vi "Test SG02P2 und G05P1.vi"() -> ()   [LabVIEW 2009]
uses:
  LV-BME Interface/ChnlSettings.ctl
  LV-BME Interface/BME_DG_TriggerSettings.ctl
  DG Classes/BME_DG_System/UpdateChnlTask.ctl
  DG Classes/BME_DG_G05P2/SG05P2 Clock and Trigger Settings.ctl
  LV-BME Interface/ClockSource.ctl
  DG Classes/BME_DG_System/BME_DG_System.lvclass
  ChnlParam.ctl
  DG Classes/BME_DG_Base/BME_DG_Base.lvclass
  DG Classes/BME_DG_Chnl/BME_DG_Chnl.lvclass
  POLARIS BME DG.lvlib
panel:
  in  "Karten Parameter":T1[](array[typedef])=[{"Trigger"={"InputTerminated?"=FALSE, "InternalClockPeriode(µs)"=1000000.0, "TriggerLevel"=1.25, "PresetValue"=0, "DivideBy"=1, "Clock Source"=1, "Gate Divider"=1, "PositiveGate?"=TRUE, "InternalTrigger?"=TRUE, "InternalArm?"=FALSE, "SWTrigger?"=FALSE, "RisingEdge?"=FALSE, "StopOnPreset?"=FALSE, "ResetWhenDone?"=TRUE, "TriggerEnabled?"=TRUE}, "ClockSource "=1, "V2 Trigger"={"Gate Type"=TRUE, "Synchronize Gate"=FALSE, "Force Trigger (µs)"=0.0, "MS Bus"=16}, " prescaller crst oscill."=8, "CardName"="Master"}, {"Trigger"={"InputTerminated?"=TRUE, "InternalClockPeriode(µs)"=0.0, "TriggerLevel"=1.25, "PresetValue"=0, "DivideBy"=1, "Clock Source"=3, "Gate Divider"=1, "PositiveGate?"=TRUE, "InternalTrigger?"=FALSE, "InternalArm?"=FALSE, "SWTrigger?"=FALSE, "RisingEdge?"=FALSE, "StopOnPreset?"=FALSE, "ResetWhenDone?"=FALSE, "TriggerEnabled?"=FALSE}, "ClockSource "=4, "V2 Trigger"={"Gate Type"=TRUE, "Synchronize Gate"=FALSE, "Force Trigger (µs)"=0.0, "MS Bus"=16}, " prescaller crst oscill."=1, "CardName"="S1"}, {"Trigger"={"InputTerminated?"=TRUE, "InternalClockPeriode(µs)"=0.0, "TriggerLevel"=1.25, "PresetValue"=0, "DivideBy"=1, "Clock Source"=3, "Gate Divider"=1, "PositiveGate?"=TRUE, "InternalTrigger?"=FALSE, "InternalArm?"=FALSE, "SWTrigger?"=FALSE, "RisingEdge?"=FALSE, "StopOnPreset?"=FALSE, "ResetWhenDone?"=FALSE, "TriggerEnabled?"=TRUE}, "ClockSource "=1, "V2 Trigger"={"Gate Type"=TRUE, "Synchronize Gate"=FALSE, "Force Trigger (µs)"=0.0, "MS Bus"=16}, " prescaller crst oscill."=1, "CardName"="S2"}] {"V2 Trigger"."MS Bus" format="%04x" items=["Local Primary"=1, "Local Secondary"=2, "Local Force"=4, "Resynchronize"=8, "Master Primary"=16, "Master Secondary"=32, "Master Force"=64, "System Clock"=128, "Delay Clock"=256, "Inhibit Local"=512, "Start Local"=1024, "Start Bus"=2048, "Step Back Local"=4096, "Step Back Bus"=8192, "Enable From E"=65536, "Enable From F"=131072, "Enable From Bus"=262144]; "V2 Trigger"."Force Trigger (µs)" min=0.0 format="%.6f"; "ClockSource" items=["Internal Oscillator"=1, "External Trigger"=2, "Trigger & Oscillator"=3, "MasterSlave Bus"=4]; "Trigger"."Gate Divider" min=1 max=1000000; "Trigger"."Clock Source" items=["Internal Oscillator"=1, "External Trigger"=2, "Trigger & Oscillator"=3]; "Trigger"."InternalClockPeriode(µs)" format="%#_11g"}
  out "Problem Chnls out":string[](array[string])
  out "DelayFormulas":string[](array[string])
  in  "Reset Error":bool
  out "error out":errorcluster
  in  "Update Delay formula":bool=TRUE
  in  "DelayFormula":string="MasterSG02P2_ChnlT0 + 100"
  in  "Aknowledge interrupts":bool
  in  "stop 3":bool=TRUE
  in  "SetDelay":bool=TRUE
  in  "UpdateChnl":bool=TRUE
  in  "ChnlParameter":T4 {"ChnParam2write"."Delay (µs)" min=0.0 max=100000000.0 format="%.5f"}
  out "CountsRemains":i32
  out "TriggerCounters":i32[](array[numeric])
  out "Interrupts":u32[](array[numeric]) format="%b"
  out "RemainingTriggers":T6(array[cluster])=[[{"Time Stamp"=timestamp(3416308194.6875 s since 1904-01-01), "Numeric"=-64}, {"Time Stamp"=timestamp(3416308194.6875 s since 1904-01-01), "Numeric"=4}, {"Time Stamp"=timestamp(3416308194.6875 s since 1904-01-01), "Numeric"=-64}, {"Time Stamp"=timestamp(3416308194.6875 s since 1904-01-01), "Numeric"=-64}], [{"Time Stamp"=timestamp(3416308194.6875 s since 1904-01-01), "Numeric"=-64}, {"Time Stamp"=timestamp(3416308194.6875 s since 1904-01-01), "Numeric"=-64}, {"Time Stamp"=timestamp(3416308194.6875 s since 1904-01-01), "Numeric"=-64}, {"Time Stamp"=timestamp(3416308194.6875 s since 1904-01-01), "Numeric"=-64}], [{"Time Stamp"=timestamp(3416308194.6875 s since 1904-01-01), "Numeric"=-64}, {"Time Stamp"=timestamp(3416308194.6875 s since 1904-01-01), "Numeric"=-64}, {"Time Stamp"=timestamp(3416308194.6875 s since 1904-01-01), "Numeric"=-64}, {"Time Stamp"=timestamp(3416308194.6875 s since 1904-01-01), "Numeric"=-64}]] {"Time Stamp" format="%<%I:%M:%S%3u %p>T"}
  in  "stop 2":bool=TRUE
  in  "ReadStatus":bool=TRUE
  in  "Activate":bool
  in  "ResetModuloCounters":bool=TRUE
  in  "TriggerModulo":u32=4
  out "Modulo Settings":u32[](array[numeric])
  out "Chnls":T5[](array[typedef])=[{" Delay (µs)"=0.0, "On? (false)"=TRUE, "PositiveVoltage?"=TRUE, "50OhmTerminated? "=TRUE, "25OhmOutput?"=FALSE}, {" Delay (µs)"=0.0, "On? (false)"=TRUE, "PositiveVoltage?"=TRUE, "50OhmTerminated? "=TRUE, "25OhmOutput?"=FALSE}, {" Delay (µs)"=0.0, "On? (false)"=TRUE, "PositiveVoltage?"=TRUE, "50OhmTerminated? "=TRUE, "25OhmOutput?"=FALSE}] {"Delay (µs)" min=0.0 max=100000000.0 format="%.5f"}
  in  "Trigger Base":T2={"InputTerminated?"=FALSE, "InternalClockPeriode(µs)"=1000000.0, "TriggerLevel"=1.25, "PresetValue"=0, "DivideBy"=1, "Clock Source"=1, "Gate Divider"=1, "PositiveGate?"=TRUE, "InternalTrigger?"=FALSE, "InternalArm?"=FALSE, "SWTrigger?"=FALSE, "RisingEdge?"=FALSE, "StopOnPreset?"=FALSE, "ResetWhenDone?"=TRUE, "TriggerEnabled?"=TRUE} {"Gate Divider" min=1 max=1000000; "Clock Source" items=["Internal Oscillator"=1, "External Trigger"=2, "Trigger & Oscillator"=3]; "InternalClockPeriode(µs)" format="%#_11g"}
  in  "Selected Chnl":u16(ring) items=["T2", "A2", "B2"]
  in  "Selected Card":u16(ring)=1 items=["Master", "S1", "S2"]
  in  "STOP":bool=TRUE
  in  "ChnParam2write":T5={" Delay (µs)"=0.0, "On? (false)"=TRUE, "PositiveVoltage?"=TRUE, "50OhmTerminated? "=TRUE, "25OhmOutput?"=FALSE} {"Delay (µs)" min=0.0 max=100000000.0 format="%.5f"}
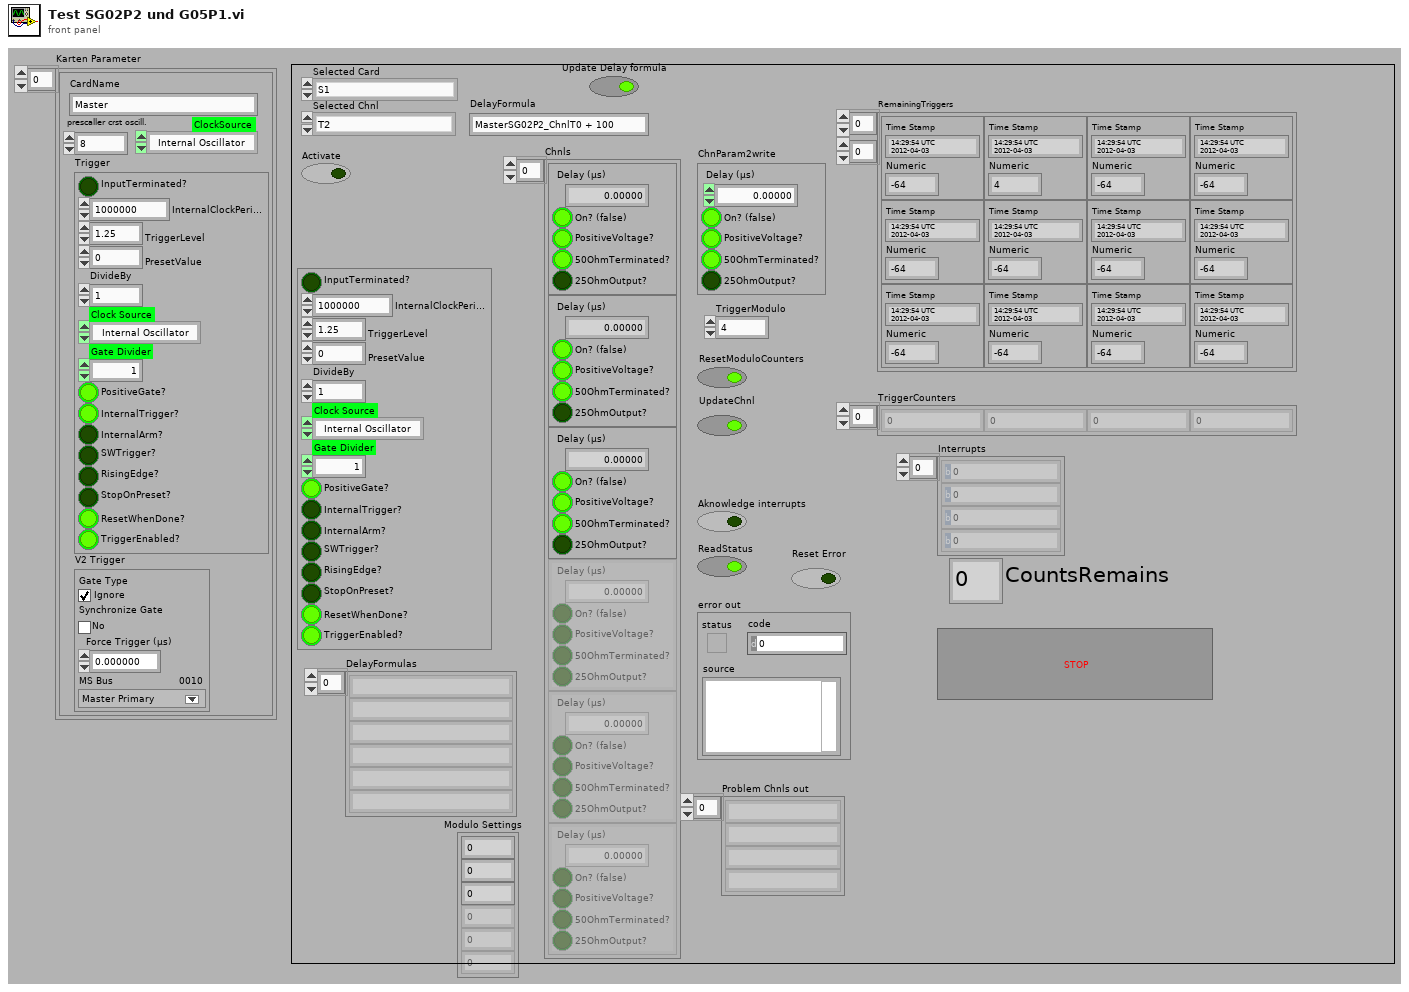
[diagram p1: front panel]
types:
  T1 = typedef "SG05P2 Clock and Trigger Settings.ctl" = cluster{"Trigger":T2, "ClockSource ":T3, "V2 Trigger":cluster{"Gate Type":bool, "Synchronize Gate":bool, "Force Trigger (µs)":dbl, "MS Bus":u32}, " prescaller crst oscill.":u32, "CardName":string}
  T2 = typedef "POLARIS BME DG.lvlib/BME_DG_TriggerSettings.ctl" = cluster{"InputTerminated?":bool, "InternalClockPeriode(µs)":dbl, "TriggerLevel":dbl, "PresetValue":i32, "DivideBy":i32, "Clock Source":u32, "Gate Divider":i32, "PositiveGate?":bool, "InternalTrigger?":bool, "InternalArm?":bool, "SWTrigger?":bool, "RisingEdge?":bool, "StopOnPreset?":bool, "ResetWhenDone?":bool, "TriggerEnabled?":bool}
  T3 = typedef "POLARIS BME DG.lvlib/ClockSource.ctl" = i32
  T4 = typedef "POLARIS BME DG.lvlib/UpdateChnlTask.ctl" = cluster{"ChnlName":string, "ChnParam2write":T5, "TriggerModulo":u32}
  T5 = typedef "POLARIS BME DG.lvlib/ChnlSettings.ctl" = cluster{" Delay (µs)":dbl, "On? (false)":bool, "PositiveVoltage?":bool, "50OhmTerminated? ":bool, "25OhmOutput?":bool}
  T6 = cluster{"Time Stamp":timestamp, "Numeric":i32}[][]
  T7 = typedef "ChnlParam.ctl" = cluster{"ChnlName":string, "DelayFormula":string, "OutputModulo":i32}
  T8 = enum8{"Enabled", "Disabled", "Disabled and Grayed Out"}
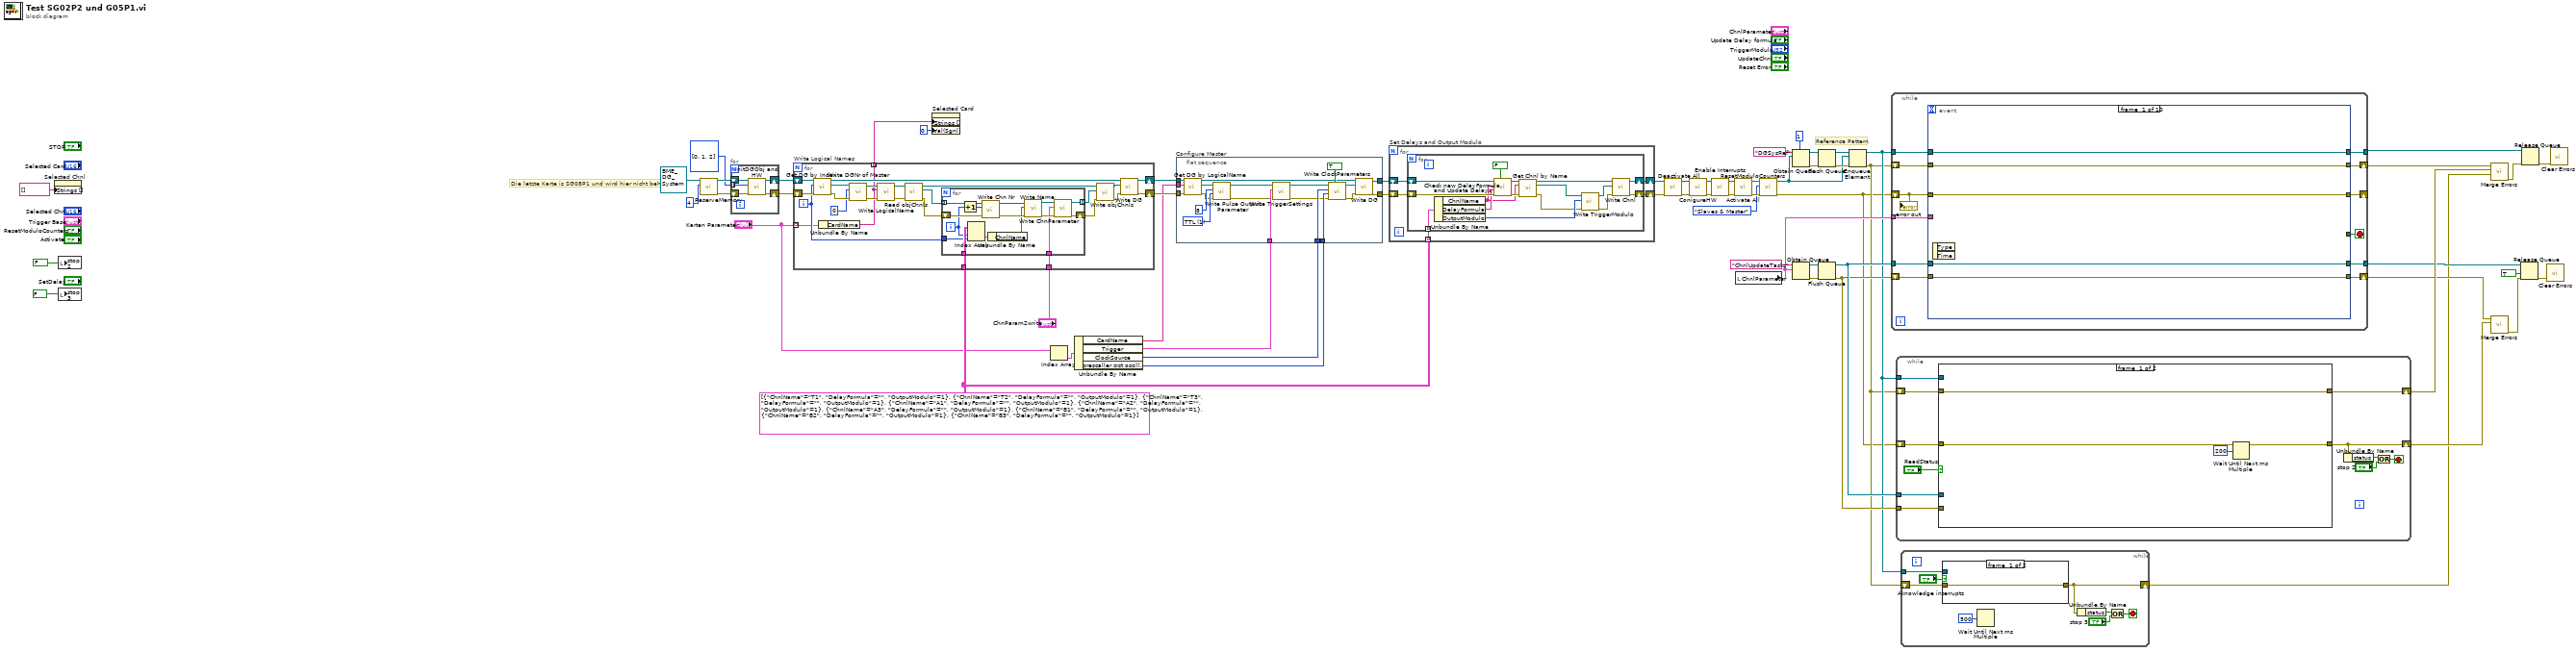
[diagram p0: block diagram]
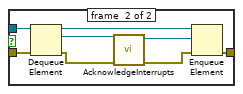
[diagram p2: hidden frame]
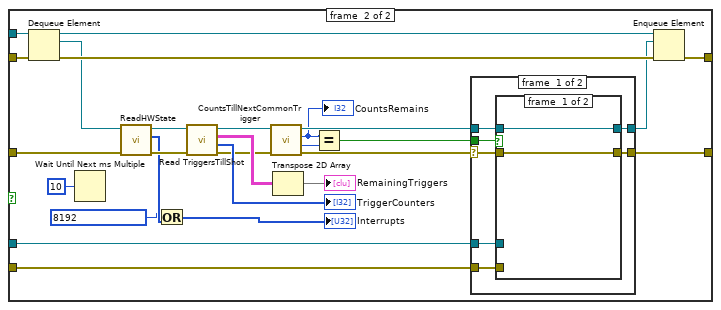
[diagram p3: hidden frame]
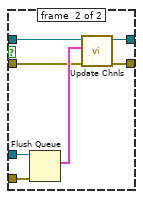
[diagram p4: hidden frame]
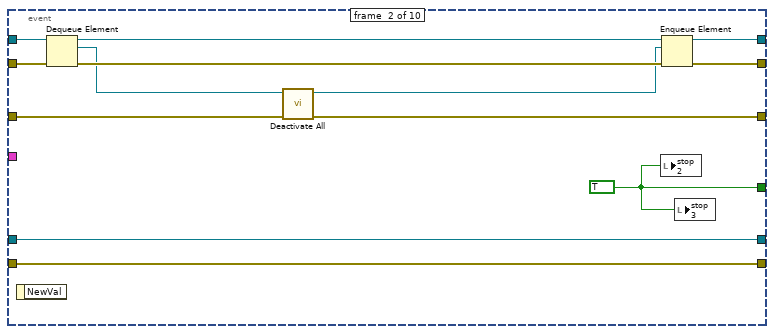
[diagram p6: hidden frame]
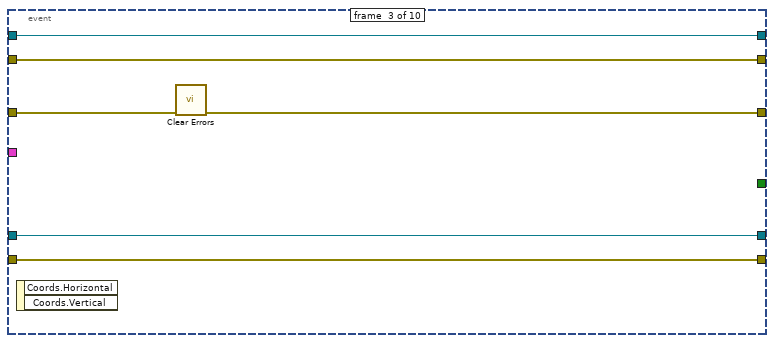
[diagram p7: hidden frame]
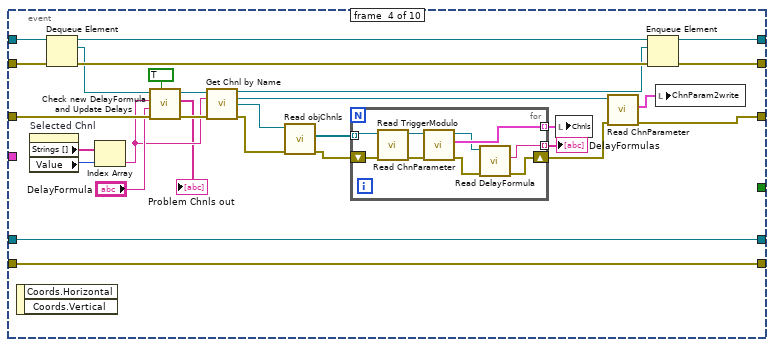
[diagram p8: hidden frame]
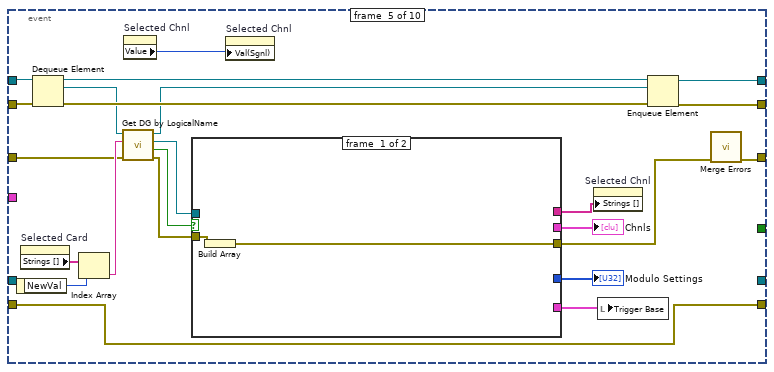
[diagram p9: hidden frame]
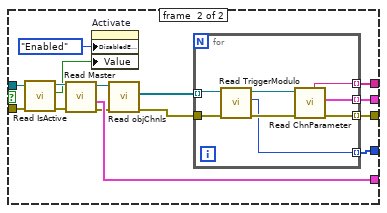
[diagram p10: hidden frame]
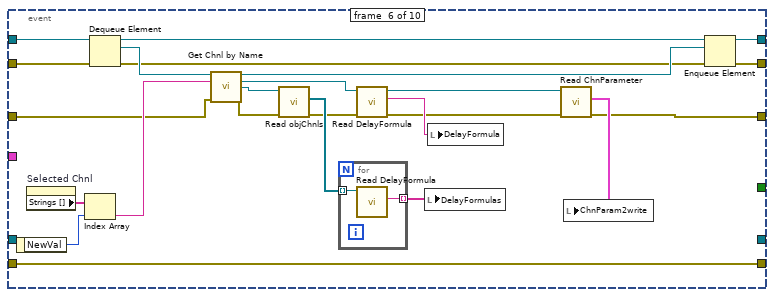
[diagram p11: hidden frame]
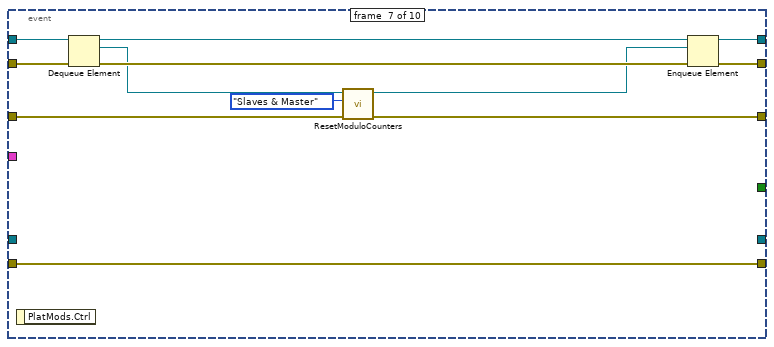
[diagram p12: hidden frame]
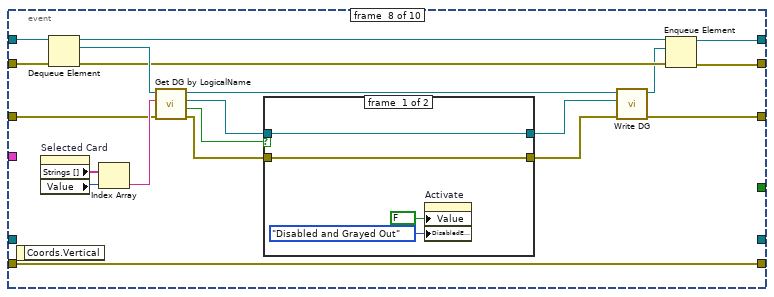
[diagram p13: hidden frame]
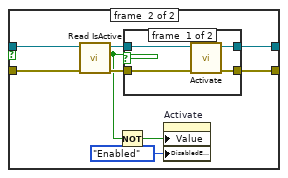
[diagram p14: hidden frame]
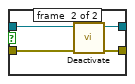
[diagram p15: hidden frame]
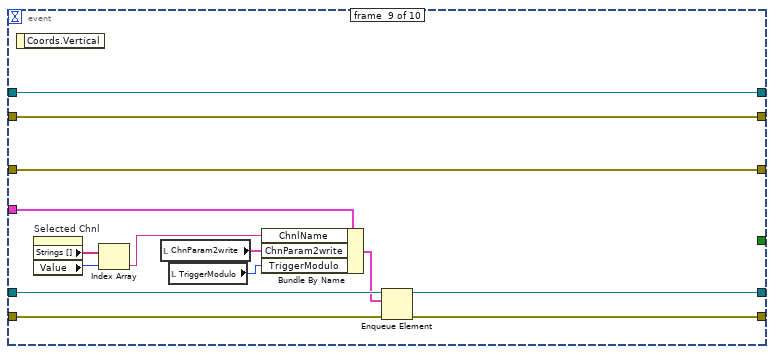
[diagram p16: hidden frame]
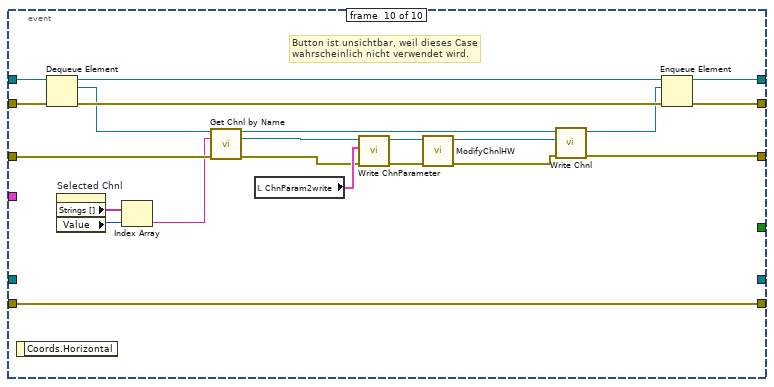
[diagram p17: hidden frame]
diagram:
  w20 = T7[][] [[{"ChnlName"="T1", "DelayFormula"="", "OutputModulo"=1}, {"ChnlName"="T2", "DelayFormula"="", "OutputModulo"=1}, {"ChnlName"="T3", "DelayFormula"="", "OutputModulo"=1}], [{"ChnlName"="A1", "DelayFormula"="", "OutputModulo"=1}, {"ChnlName"="A2", "DelayFormula"="", "OutputModulo"=1}, {"ChnlName"="A3", "DelayFormula"="", "OutputModulo"=1}], [{"ChnlName"="B1", "DelayFormula"="", "OutputModulo"=1}, {"ChnlName"="B2", "DelayFormula"="", "OutputModulo"=1}, {"ChnlName"="B3", "DelayFormula"="", "OutputModulo"=1}]] ("ChnlParam 2")
  # "Die letzte Karte is SG08P1 und wird hier nicht behandelt"
  # "Reference Pattern"
  n1 = property on="Selected Chnl" class="Ring (strict)"("Strings []"=string[] []) -> ()  [unwired: 2 in, 2 out]
  n2 = local write "stop 2"(FALSE ("stop 2")) -> ()
  n3 = local write "stop 3"(FALSE ("stop 3")) -> ()
  n4 = call "ReserveMemory.vi"("#DGs"=4, "BME_DG_System in"=refnum<class "BME_DG_System.lvclass"> refnum ("BME_DG_System.lvclass")) -> ("error out"=w6:errorcluster, "BME_DG_System out"=w7:refnum<class "BME_DG_System.lvclass">)  [unwired: 8 in]
  n5 = for {
    tunnel: i32[] [0, 1, 2] -> [w64] mode=indexing
    shift-right: [w66] -> w3
    shift-left: w7 -> [w68]
    shift-right: [w65] -> w2
    shift-left: w6 -> [w67]
    n6 = call "InitDGObj and HW.vi"("error out"=w67, "DGNr"=w64, "BME_DG_System in"=w68) -> ("error IO"=w65:errorcluster, "BME_DG_System Out"=w66:refnum<class "BME_DG_System.lvclass">)  [unwired: 3 in]
  }
  n7 = for "Write Logical Names" {
    shift-right: [w89] -> w19
    shift-left: w3 -> [w92]
    shift-right: [w88] -> w16
    shift-left: w2 -> [w91]
    tunnel: "ChnParam2write" -> [w85]
    tunnel: w20 -> [w81]
    tunnel: [w72] -> w38 mode=indexing
    tunnel: "Karten Parameter" -> [w73] mode=indexing
    i -> [w74]
    n8 = call "Get DG by Index.vi"("error in (no error)"=w91, "index"=w74, "BME_DG_System in"=w92) -> ("error out"=w75:errorcluster, "BME_DG_Base.lvclass"=w78:refnum<class "BME_DG_Base.lvclass">, "BME_DG_System out"=w90:refnum<class "BME_DG_System.lvclass">)  [unwired: 6 in]
    n9 = Unbundle By Name(w73) -> ("CardName"=w72:string)
    n10 = call-dynamic "Write DGNr of Master.vi"("error in (no error)"=w75, "DGNr of Master"=0, "BME_DG_Base in"=w78) -> ("error out"=w76:errorcluster, "BME_DG_Base out"=w77:refnum<class "BME_DG_Base.lvclass">)  [unwired: 7 in]
    n11 = call "Write LogicalName.vi"("error in (no error)"=w76, "LogicalName"=w72, "BME_DG_Base in"=w77) -> ("error out"=w79:errorcluster, "BME_DG_Base out"=w80:refnum<class "BME_DG_Base.lvclass">)  [unwired: 7 in]
    n12 = call-dynamic "Read objChnls.vi"("error in (no error)"=w79, "BME_DG_Base in"=w80) -> ("error out"=w86:errorcluster, "objChnls"=w87:refnum<class "BME_DG_Chnl.lvclass">[], "BME_DG_Base out"=w83:refnum<class "BME_DG_Base.lvclass">)  [unwired: 6 in, 1 out]
    n13 = for {
      tunnel: w87 -> [w104] mode=indexing
      shift-right: [w96] -> w82
      shift-left: w86 -> [w102]
      tunnel: w85 -> [w105]
      tunnel: [w97] -> w84 mode=indexing
      tunnel: w81 -> [w99]
      tunnel: w74 -> [w94]
      i -> [w95]
      n14 = Increment(x=w95) -> (x+1=w100:i32)
      n15 = Index Array(array=w99, index (row)=w95, index (col)=w94) -> (element=w98:T7)
      n16 = call-dynamic "Write Chn Nr.vi"("error in (no error)"=w102, "Chn Nr"=w100, "BME_DG_Chnl in"=w104) -> ("error out"=w101:errorcluster, "BME_DG_Chnl out"=w103:refnum<class "BME_DG_Chnl.lvclass">)  [unwired: 7 in]
      n17 = Unbundle By Name(w98) -> ("ChnlName"=w93:string)
      n18 = call-dynamic "Write Name.vi"("error in (no error)"=w101, "Name"=w93, "BME_DG_Chnl in"=w103) -> ("error out"=w106:errorcluster, "BME_DG_Chnl out"=w107:refnum<class "BME_DG_Chnl.lvclass">)  [unwired: 7 in]
      n19 = call-dynamic "Write ChnParameter.vi"("error in (no error)"=w106, "ChnParemater"=w105, "BME_DG_Chnl in"=w107) -> ("error out"=w96:errorcluster, "BME_DG_Chnl out"=w97:refnum<class "BME_DG_Chnl.lvclass">)  [unwired: 7 in]
    }
    n20 = call-dynamic "Write objChnls.vi"("error in (no error)"=w82, "objChnls"=w84, "BME_DG_Base in"=w83) -> ("error out"=w71:errorcluster, "BME_DG_Base out"=w70:refnum<class "BME_DG_Base.lvclass">)  [unwired: 7 in]
    n21 = call "Write DG.vi"("error in (no error)"=w71, "BME_DG_Base"=w70, "BME_DG_System in"=w90) -> ("error out"=w88:errorcluster, "BME_DG_System out"=w89:refnum<class "BME_DG_System.lvclass">)  [unwired: 7 in]
  }
  n22 = property on="Selected Card" class="Ring (strict)"("Strings []"=w38, "Val(Sgnl)"=u16 0 ("Value (Signaling)")) -> ()  [unwired: 2 in, 2 out]
  n23 = Index Array(array="Karten Parameter") -> (element=w14:T1)  [unwired: 1 in]
  n24 = Unbundle By Name(w14) -> ("CardName"=w13:string, "Trigger"=w12:T2, "ClockSource"=w10:T3, "prescaller crst oscill."=w11:u32)
  n25 = flat-sequence "Configure Master" {
    tunnel: w19 -> [w124]
    tunnel: [w123] -> w18
    tunnel: [w122] -> w17
    tunnel: w16 -> [w121]
    tunnel: w13 -> [w120]
    tunnel: w12 -> [w115]
    tunnel: w10 -> [w114]
    tunnel: w11 -> [w113]
    frame #0 {
      w126 = u32 1 items=["TTL"=1, "NIM"=2, "ECL"=3] ("Pulse Output Level")
      n26 = call "Get DG by LogicalName.vi"("error in (no error)"=w121, "LogicalName"=w120, "BME_DG_System in"=w124) -> ("error out"=w117:errorcluster, "BME_DG_Base.lvclass"=w119:refnum<class "BME_DG_Base.lvclass">, "BME_DG_System out"=w112:refnum<class "BME_DG_System.lvclass">)  [unwired: 5 in, 1 out]
      n27 = call-dynamic "Write Pulse Output Parameter.vi"("error in (no error)"=w117, "Pulse Output Level"=w126, "Pulse Width"=u32 8, "BME_DG_Base in"=w119) -> ("error out"=w110:errorcluster, "BME_DG_Base out"=w111:refnum<class "BME_DG_Base.lvclass">)  [unwired: 6 in]
      n28 = call-dynamic "Write TriggerSettings.vi"("error in (no error)"=w110, "Trigger Settings"=w115, "BME_DG_Base in"=w111) -> ("error out"=w109:errorcluster, "BME_DG_Base out"=w108:refnum<class "BME_DG_Base.lvclass">)  [unwired: 7 in]
      n29 = call-dynamic "Write ClockParameters.vi"("ClockEnable"=TRUE, "error in (no error)"=w109, "PrescalerCrystalOscilator"=w113, "ClockSource"=w114, "BME_DG_Base in"=w108) -> ("error out"=w116:errorcluster, "BME_DG_Base out"=w118:refnum<class "BME_DG_Base.lvclass">)  [unwired: 5 in]
      n30 = call "Write DG.vi"("error in (no error)"=w116, "BME_DG_Base"=w118, "BME_DG_System in"=w112) -> ("error out"=w122:errorcluster, "BME_DG_System out"=w123:refnum<class "BME_DG_System.lvclass">)  [unwired: 7 in]
    }
  }
  n31 = for "Set Delays and Output Modulo" {
    shift-right: [w131] -> w22
    shift-left: w18 -> [w132]
    shift-right: [w129] -> w21
    shift-left: w17 -> [w130]
    tunnel: w20 -> [w128] mode=indexing
    n32 = for {
      shift-right: [w139] -> w131
      shift-left: w132 -> [w148]
      shift-right: [w138] -> w129
      shift-left: w130 -> [w147]
      tunnel: w128 -> [w145] mode=indexing
      n33 = Unbundle By Name(w145) -> ("ChnlName"=w141:string, "DelayFormula"=w144:string, "OutputModulo"=w140:i32)
      n34 = call "Check new DelayFormula and Update Delays.vi"("Update HW"=FALSE, "error in (no error)"=w147, "Delay Formula"=w144, "ChnlName"=w141, "BME_DG_System in"=w148) -> ("error out"=w142:errorcluster, "BME_DG_System out"=w143:refnum<class "BME_DG_System.lvclass">)  [unwired: 4 in, 1 out]
      n35 = call "Get Chnl by Name.vi"("BME_DG_System in"=w143, "Chnl Name"=w141, "error in (no error)"=w142) -> ("BME_DG_System out"=w137:refnum<class "BME_DG_System.lvclass">, "BME_DG_Chnl"=w133:refnum<class "BME_DG_Chnl.lvclass">, "error out"=w134:errorcluster)  [unwired: 7 in, 3 out]
      n36 = call-dynamic "Write TriggerModulo.vi"("error in (no error)"=w134, "TriggerModulo"=w140, "BME_DG_G05_Chnl in"=w133) -> ("error out"=w136:errorcluster, "BME_DG_G05_Chnl out"=w135:refnum<class "BME_DG_Chnl.lvclass">)  [unwired: 7 in]
      n37 = call "Write Chnl.vi"("error in (no error)"=w136, "BME_DG_Chnl.lvclass"=w135, "BME_DG_System in"=w137) -> ("error out"=w138:errorcluster, "BME_DG_System out"=w139:refnum<class "BME_DG_System.lvclass">)  [unwired: 7 in]
    }
  }
  n38 = call "Deactivate All.vi"("error in (no error)"=w21, "BME_DG_System in"=w22) -> ("error out"=w36:errorcluster, "BME_DG_System out"=w37:refnum<class "BME_DG_System.lvclass">)  [unwired: 8 in]
  n39 = call "ConigureHW.vi"("error in (no error)"=w36, "BME_DG_System in"=w37) -> ("error out"=w34:errorcluster, "BME_DG_System out"=w35:refnum<class "BME_DG_System.lvclass">)  [unwired: 8 in]
  n40 = call "Enable Interrupts.vi"("error in (no error)"=w34, "BME_DG_System in"=w35) -> ("error out"=w28:errorcluster, "BME_DG_System out"=w29:refnum<class "BME_DG_System.lvclass">)  [unwired: 8 in]
  n41 = call "Activate All.vi"("error in (no error)"=w28, "BME_DG_System in"=w29) -> ("error out"=w25:errorcluster, "BME_DG_System out"=w27:refnum<class "BME_DG_System.lvclass">)  [unwired: 8 in]
  n42 = local read "ChnlParameter"() -> (w46:T4)
  n43 = call "ResetModuloCounters.vi"("error in (no error)"=w25, "Enum"=enum16{"Slaves only", "Slaves & Master"}."Slaves & Master", "BME_DG_System in"=w27) -> ("error out"=w24:errorcluster, "BME_DG_System out"=w26:refnum<class "BME_DG_System.lvclass">)  [unwired: 7 in]
  n44 = Obtain Queue(max queue size (-1, unlimited)=1, name (unnamed)="DGSysRef", element data type=w26) -> (queue out=w54:refnum<queue>, error out=w52:errorcluster)  [unwired: 2 in, 1 out]
  n45 = Obtain Queue(name (unnamed)="ChnlUpdateTasks", element data type=w46) -> (queue out=w47:refnum<queue>, error out=w48:errorcluster)  [unwired: 3 in, 1 out]
  n46 = Flush Queue(queue=w54, error in (no error)=w52) -> (queue out=w53:refnum<queue>, error out=w51:errorcluster)  [unwired: 1 out]
  n47 = Flush Queue(queue=w47, error in (no error)=w48) -> (queue out=w43:refnum<queue>, error out=w42:errorcluster)  [unwired: 1 out]
  n48 = Enqueue Element(queue=w53, element=w26, error in (no error)=w51) -> (queue out=w33:refnum<queue>, error out=w32:errorcluster)  [unwired: 1 in, 1 out]
  n49 = while {
    shift-right: [w156] -> _
    shift-left: w24 -> [w158]
    shift-right: [w154] -> w57
    shift-left: w32 -> [w155]
    tunnel: w33 -> [w159]
    tunnel: [w157] -> w59
    tunnel: w43 -> [w153]
    tunnel: w46 -> [w152]
    tunnel: [w150] -> w45
    shift-right: [w149] -> w41
    shift-left: w42 -> [w151]
    stop <- w160 stop-if-true
    n50 = event shown="[3] \"Update Delay formula\": Mouse Down" {
      selector: _ -> [_ _ _ _ _ _ _ _ _ _]
      dyn-events: _ -> [_ _ _ _ _ _ _ _ _ _]
      timeout: _ -> [_ _ _ _ _ _ _ _ _ _]
      tunnel: [_ w166 _ _ _ _ _ _ _ _] -> w160
      tunnel: w159 -> [w165 w175 w183 w212 w233 w290 w308 w317 w363 w384]
      tunnel: w158 -> [w164 w178 w184 w204 w242 w274 w298 w325 w362 w375]
      tunnel: [w165 w171 w183 w208 w231 w288 w303 w311 w363 w380] -> w157
      tunnel: [w164 w177 w179 w187 w226 w271 w299 w318 w362 w364] -> w156
      tunnel: w155 -> [w163 w174 w182 w211 w232 w289 w306 w316 w359 w383]
      tunnel: [w163 w172 w182 w209 w230 w287 w304 w310 w359 w381] -> w154
      tunnel: w153 -> [w162 w168 w181 w207 _ _ _ _ w354 _]
      tunnel: w152 -> [_ _ _ _ _ _ _ _ w358 _]
      tunnel: w151 -> [w161 w167 w180 w206 w224 w294 w302 w309 w352 w379]
      tunnel: [w162 w168 w181 w207 _ _ _ _ w351 _] -> w150
      tunnel: [w161 w167 w180 w206 w224 w294 w302 w309 w350 w379] -> w149
      event #0 {
        n51 = event-data() -> ()  [unwired: 1 in, 2 out]
      }
      event #1 {
        w166 = TRUE
        n52 = event-data() -> ()  [unwired: 1 in, 1 out]
        n53 = Dequeue Element(queue=w175, error in (no error)=w174) -> (queue out=w176:refnum<queue>, element=w169:refnum<class "BME_DG_System.lvclass">, error out=w173:errorcluster)  [unwired: 1 in, 1 out]
        n54 = call "Deactivate All.vi"("error in (no error)"=w178, "BME_DG_System in"=w169) -> ("error out"=w177:errorcluster, "BME_DG_System out"=w170:refnum<class "BME_DG_System.lvclass">)  [unwired: 8 in]
        n55 = local write "stop 2"(w166) -> ()
        n56 = Enqueue Element(queue=w176, element=w170, error in (no error)=w173) -> (queue out=w171:refnum<queue>, error out=w172:errorcluster)  [unwired: 1 in, 1 out]
        n57 = local write "stop 3"(w166) -> ()
      }
      event #2 {
        n58 = event-data() -> ()  [unwired: 1 in, 2 out]
        n59 = call <vilib>:"Clear Errors.vi"("error in (no error)"=w184) -> ("error out"=w179:errorcluster)  [unwired: 6 in]
      }
      event #3 {
        n60 = event-data() -> ()  [unwired: 1 in, 2 out]
        n61 = property on="Selected Chnl" class="Ring (strict)"() -> ("Strings []"=w202:string[], "Value"=w203:u16)  [unwired: 2 in, 2 out]
        n62 = Dequeue Element(queue=w212, error in (no error)=w211) -> (queue out=w213:refnum<queue>, element=w205:refnum<class "BME_DG_System.lvclass">, error out=w210:errorcluster)  [unwired: 1 in, 1 out]
        n63 = Index Array(array=w202, index=w203) -> (element=w192:string)
        n64 = call "Check new DelayFormula and Update Delays.vi"("Update HW"=TRUE, "error in (no error)"=w204, "Delay Formula"="DelayFormula", "ChnlName"=w192, "BME_DG_System in"=w205) -> ("error out"=w194:errorcluster, "Problem Chnls out"=→"Problem Chnls out":string[], "BME_DG_System out"=w196:refnum<class "BME_DG_System.lvclass">)  [unwired: 4 in]
        n65 = call "Get Chnl by Name.vi"("BME_DG_System in"=w196, "Chnl Name"=w192, "error in (no error)"=w194) -> ("BME_DG_System out"=w195:refnum<class "BME_DG_System.lvclass">, "BME_DG_Chnl"=w189:refnum<class "BME_DG_Chnl.lvclass">, "Owner DG"=w197:refnum<class "BME_DG_Base.lvclass">, "error out"=w193:errorcluster)  [unwired: 7 in, 2 out]
        n66 = call-dynamic "Read objChnls.vi"("error in (no error)"=w193, "BME_DG_Base in"=w197) -> ("error out"=w198:errorcluster, "objChnls"=w200:refnum<class "BME_DG_Chnl.lvclass">[])  [unwired: 6 in, 2 out]
        n67 = for {
          tunnel: w200 -> [w221] mode=indexing
          tunnel: [w222] -> w199 mode=indexing
          shift-right: [w214] -> w188
          shift-left: w198 -> [w219]
          tunnel: [w215] -> w191 mode=indexing
          n68 = call-dynamic "Read TriggerModulo.vi"("error in (no error)"=w219, "BME_DG_Chnl in"=w221) -> ("error out"=w218:errorcluster, "BME_DG_Chnl out"=w220:refnum<class "BME_DG_Chnl.lvclass">)  [unwired: 7 in, 1 out]
          n69 = call-dynamic "Read ChnParameter.vi"("error in (no error)"=w218, "BME_DG_Chnl in"=w220) -> ("error out"=w216:errorcluster, "ChnParemater"=w222:T5, "BME_DG_Chnl out"=w217:refnum<class "BME_DG_Chnl.lvclass">)  [unwired: 4 in, 3 out]
          n70 = call-dynamic "Read DelayFormula.vi"("error in (no error)"=w216, "BME_DG_Chnl in"=w217) -> ("error out"=w214:errorcluster, "DelayFormula"=w215:string)  [unwired: 7 in, 1 out]
        }
        "DelayFormulas" <- w191
        n71 = local write "Chnls"(w199) -> ()
        n72 = call-dynamic "Read ChnParameter.vi"("error in (no error)"=w188, "BME_DG_Chnl in"=w189) -> ("error out"=w187:errorcluster, "ChnParemater"=w186:T5)  [unwired: 4 in, 4 out]
        n73 = Enqueue Element(queue=w213, element=w195, error in (no error)=w210) -> (queue out=w208:refnum<queue>, error out=w209:errorcluster)  [unwired: 1 in, 1 out]
        n74 = local write "ChnParam2write"(w186) -> ()
      }
      event #4 {
        n75 = event-data() -> ("NewVal"=w244:u16)  [unwired: 1 in]
        n76 = property on="Selected Card" class="Ring (strict)"() -> ("Strings []"=w245:string[])  [unwired: 2 in, 2 out]
        n77 = Dequeue Element(queue=w233, error in (no error)=w232) -> (queue out=w234:refnum<queue>, element=w229:refnum<class "BME_DG_System.lvclass">, error out=w235:errorcluster)  [unwired: 1 in, 1 out]
        n78 = Index Array(array=w245, index=w244) -> (element=w243:string)
        n79 = call "Get DG by LogicalName.vi"("error in (no error)"=w242, "LogicalName"=w243, "BME_DG_System in"=w229) -> ("error out"=w227:errorcluster, "found?"=w241:bool, "BME_DG_Base.lvclass"=w240:refnum<class "BME_DG_Base.lvclass">, "BME_DG_System out"=w228:refnum<class "BME_DG_System.lvclass">)  [unwired: 5 in]
        n80 = property on="Selected Chnl" class="Ring (strict)"() -> ("Value"=w223:u16)  [unwired: 2 in, 2 out]
        n81 = case shown="True" w241 {
          tunnel: w240 -> [_ w255]
          tunnel: [_ w262] -> w239
          tunnel: [_ w261] -> w237
          tunnel: [_ w260] -> w238
          tunnel: [_ w256] -> w236
          tunnel: w227 -> [w247 w252]
          tunnel: [w246 w250] -> w225
          frame #0 {
            n82 = Build Array(w247) -> (w246:errorcluster[])
          }
          frame #1 {
            n83 = call-dynamic "Read IsActive.vi"("error in (no error)"=w252, "BME_DG_Base in"=w255) -> ("error out"=w253:errorcluster, "Active?"=w248:bool, "BME_DG_Base out"=w254:refnum<class "BME_DG_Base.lvclass">)  [unwired: 7 in]
            n84 = call-dynamic "Read Master.vi"("error in (no error)"=w253, "BME_DG_Base in"=w254) -> ("error out"=w257:errorcluster, "TriggerSettings"=w260:T2, "BME_DG_Base out"=w258:refnum<class "BME_DG_Base.lvclass">)  [unwired: 6 in, 1 out]
            n85 = property on="Activate" class="Bool (strict)"("DisabledEnum"=T8."Enabled" ("Disabled"), "Value"=w248) -> ()  [unwired: 2 in, 2 out]
            n86 = call-dynamic "Read objChnls.vi"("error in (no error)"=w257, "BME_DG_Base in"=w258) -> ("error out"=w251:errorcluster, "objChnls"=w259:refnum<class "BME_DG_Chnl.lvclass">[])  [unwired: 6 in, 2 out]
            n87 = for {
              tunnel: w259 -> [w268] mode=indexing
              tunnel: [w270] -> w262 mode=indexing
              tunnel: [w269] -> w261 mode=indexing
              tunnel: [w263] -> w256 mode=indexing
              tunnel: w251 -> [w266]
              tunnel: [w264] -> w250 mode=indexing
              n88 = call-dynamic "Read TriggerModulo.vi"("error in (no error)"=w266, "BME_DG_Chnl in"=w268) -> ("error out"=w265:errorcluster, "TriggerModulo"=w263:i32, "BME_DG_Chnl out"=w267:refnum<class "BME_DG_Chnl.lvclass">)  [unwired: 7 in]
              n89 = call-dynamic "Read ChnParameter.vi"("error in (no error)"=w265, "BME_DG_Chnl in"=w267) -> ("error out"=w264:errorcluster, "ChnParemater"=w269:T5, "Name"=w270:string)  [unwired: 4 in, 3 out]
            }
          }
        }
        "Chnls" <- w237
        "Modulo Settings" <- w236
        n90 = property on="Selected Chnl" class="Ring (strict)"("Val(Sgnl)"=w223) -> ()  [unwired: 2 in, 2 out]
        n91 = property on="Selected Chnl" class="Ring (strict)"("Strings []"=w239) -> ()  [unwired: 2 in, 2 out]
        n92 = local write "Trigger Base"(w238) -> ()
        n93 = Enqueue Element(queue=w234, element=w228, error in (no error)=w235) -> (queue out=w231:refnum<queue>, error out=w230:errorcluster)  [unwired: 1 in, 1 out]
        n94 = call <vilib>:"Merge Errors.vi"("error array in"=w225) -> ("error out"=w226:errorcluster)  [unwired: 6 in]
      }
      event #5 {
        n95 = event-data() -> ("NewVal"=w292:u16)  [unwired: 1 in]
        n96 = property on="Selected Chnl" class="Ring (strict)"() -> ("Strings []"=w293:string[])  [unwired: 2 in, 2 out]
        n97 = Index Array(array=w293, index=w292) -> (element=w284:string)
        n98 = Dequeue Element(queue=w290, error in (no error)=w289) -> (queue out=w291:refnum<queue>, element=w285:refnum<class "BME_DG_System.lvclass">, error out=w275:errorcluster)  [unwired: 1 in, 1 out]
        n99 = call "Get Chnl by Name.vi"("BME_DG_System in"=w285, "Chnl Name"=w284, "error in (no error)"=w274) -> ("BME_DG_System out"=w286:refnum<class "BME_DG_System.lvclass">, "BME_DG_Chnl"=w282:refnum<class "BME_DG_Chnl.lvclass">, "Owner DG"=w281:refnum<class "BME_DG_Base.lvclass">, "error out"=w273:errorcluster)  [unwired: 7 in, 2 out]
        n100 = call-dynamic "Read objChnls.vi"("error in (no error)"=w273, "BME_DG_Base in"=w281) -> ("error out"=w272:errorcluster, "objChnls"=w280:refnum<class "BME_DG_Chnl.lvclass">[])  [unwired: 6 in, 2 out]
        n101 = for {
          tunnel: w280 -> [w296] mode=indexing
          tunnel: [w295] -> w279 mode=indexing
          n102 = call-dynamic "Read DelayFormula.vi"("BME_DG_Chnl in"=w296) -> ("DelayFormula"=w295:string)  [unwired: 8 in, 2 out]
        }
        n103 = call-dynamic "Read DelayFormula.vi"("error in (no error)"=w272, "BME_DG_Chnl in"=w282) -> ("error out"=w277:errorcluster, "DelayFormula"=w283:string, "BME_DG_Chnl out"=w276:refnum<class "BME_DG_Chnl.lvclass">)  [unwired: 7 in]
        n104 = local write "DelayFormulas"(w279) -> ()
        n105 = local write "DelayFormula"(w283) -> ()
        n106 = call-dynamic "Read ChnParameter.vi"("error in (no error)"=w277, "BME_DG_Chnl in"=w276) -> ("error out"=w271:errorcluster, "ChnParemater"=w278:T5)  [unwired: 4 in, 4 out]
        n107 = local write "ChnParam2write"(w278) -> ()
        n108 = Enqueue Element(queue=w291, element=w286, error in (no error)=w275) -> (queue out=w288:refnum<queue>, error out=w287:errorcluster)  [unwired: 1 in, 1 out]
      }
      event #6 {
        n109 = event-data() -> ()  [unwired: 1 in, 1 out]
        n110 = Dequeue Element(queue=w308, error in (no error)=w306) -> (queue out=w307:refnum<queue>, element=w301:refnum<class "BME_DG_System.lvclass">, error out=w305:errorcluster)  [unwired: 1 in, 1 out]
        n111 = call "ResetModuloCounters.vi"("error in (no error)"=w298, "Enum"=enum16{"Slaves only", "Slaves & Master"}."Slaves & Master", "BME_DG_System in"=w301) -> ("error out"=w299:errorcluster, "BME_DG_System out"=w300:refnum<class "BME_DG_System.lvclass">)  [unwired: 7 in]
        n112 = Enqueue Element(queue=w307, element=w300, error in (no error)=w305) -> (queue out=w303:refnum<queue>, error out=w304:errorcluster)  [unwired: 1 in, 1 out]
      }
      event #7 {
        n113 = event-data() -> ()  [unwired: 1 in, 1 out]
        n114 = property on="Selected Card" class="Ring (strict)"() -> ("Strings []"=w328:string[], "Value"=w327:u16)  [unwired: 2 in, 2 out]
        n115 = Dequeue Element(queue=w317, error in (no error)=w316) -> (queue out=w314:refnum<queue>, element=w315:refnum<class "BME_DG_System.lvclass">, error out=w313:errorcluster)  [unwired: 1 in, 1 out]
        n116 = Index Array(array=w328, index=w327) -> (element=w326:string)
        n117 = call "Get DG by LogicalName.vi"("error in (no error)"=w325, "LogicalName"=w326, "BME_DG_System in"=w315) -> ("error out"=w323:errorcluster, "found?"=w319:bool, "BME_DG_Base.lvclass"=w324:refnum<class "BME_DG_Base.lvclass">, "BME_DG_System out"=w320:refnum<class "BME_DG_System.lvclass">)  [unwired: 5 in]
        n118 = case shown="True" w319 {
          tunnel: w324 -> [w332 w339]
          tunnel: w323 -> [w331 w337]
          tunnel: [w331 w341] -> w322
          tunnel: [w332 w340] -> w321
          frame #0 {
            n119 = property on="Activate" class="Bool (strict)"("Value"=FALSE ("Activate"), "DisabledEnum"=T8."Disabled and Grayed Out" ("Disabled")) -> ()  [unwired: 2 in, 2 out]
          }
          frame #1 {
            n120 = call-dynamic "Read IsActive.vi"("error in (no error)"=w337, "BME_DG_Base in"=w339) -> ("error out"=w336:errorcluster, "Active?"=w335:bool, "BME_DG_Base out"=w338:refnum<class "BME_DG_Base.lvclass">)  [unwired: 7 in]
            n121 = Not(x=w335) -> (.not. x?=w333:bool)
            n122 = case shown="True" w335 {
              tunnel: [w345 w347] -> w341
              tunnel: [w344 w348] -> w340
              tunnel: w338 -> [w343 w349]
              tunnel: w336 -> [w342 w346]
              frame #0 {
                n123 = call-dynamic "Activate.vi"("error in (no error)"=w342, "BME_DG_Base in"=w343) -> ("error out"=w345:errorcluster, "BME_DG_Base out"=w344:refnum<class "BME_DG_Base.lvclass">)  [unwired: 8 in]
              }
              frame #1 {
                n124 = call-dynamic "Deactivate.vi"("error in (no error)"=w346, "BME_DG_Base in"=w349) -> ("error out"=w347:errorcluster, "BME_DG_Base out"=w348:refnum<class "BME_DG_Base.lvclass">)  [unwired: 8 in]
              }
            }
            n125 = property on="Activate" class="Bool (strict)"("Value"=w333, "DisabledEnum"=T8."Enabled" ("Disabled")) -> ()  [unwired: 2 in, 2 out]
          }
        }
        n126 = call "Write DG.vi"("error in (no error)"=w322, "BME_DG_Base"=w321, "BME_DG_System in"=w320) -> ("error out"=w318:errorcluster, "BME_DG_System out"=w312:refnum<class "BME_DG_System.lvclass">)  [unwired: 7 in]
        n127 = Enqueue Element(queue=w314, element=w312, error in (no error)=w313) -> (queue out=w311:refnum<queue>, error out=w310:errorcluster)  [unwired: 1 in, 1 out]
      }
      event #8 {
        n128 = event-data() -> ()  [unwired: 1 in, 1 out]
        n129 = property on="Selected Chnl" class="Ring (strict)"() -> ("Strings []"=w360:string[], "Value"=w361:u16)  [unwired: 2 in, 2 out]
        n130 = Index Array(array=w360, index=w361) -> (element=w357:string)
        n131 = local read "ChnParam2write"() -> (w356:T5)
        n132 = local read "TriggerModulo"() -> (w355:u32)
        n133 = Bundle By Name(cluster=w358, "ChnlName"=w357, "ChnParam2write"=w356, "TriggerModulo"=w355) -> (w353:T4)
        n134 = Enqueue Element(queue=w354, element=w353, error in (no error)=w352) -> (queue out=w351:refnum<queue>, error out=w350:errorcluster)  [unwired: 1 in, 1 out]
      }
      event #9 {
        # "Button ist unsichtbar, weil dieses Case \nwahrscheinlich nicht verwendet wird."
        n135 = event-data() -> ()  [unwired: 1 in, 1 out]
        n136 = Dequeue Element(queue=w384, error in (no error)=w383) -> (queue out=w385:refnum<queue>, element=w376:refnum<class "BME_DG_System.lvclass">, error out=w382:errorcluster)  [unwired: 1 in, 1 out]
        n137 = property on="Selected Chnl" class="Ring (strict)"() -> ("Strings []"=w377:string[], "Value"=w378:u16)  [unwired: 2 in, 2 out]
        n138 = Index Array(array=w377, index=w378) -> (element=w374:string)
        n139 = call "Get Chnl by Name.vi"("BME_DG_System in"=w376, "Chnl Name"=w374, "error in (no error)"=w375) -> ("BME_DG_System out"=w370:refnum<class "BME_DG_System.lvclass">, "BME_DG_Chnl"=w373:refnum<class "BME_DG_Chnl.lvclass">, "error out"=w371:errorcluster)  [unwired: 7 in, 3 out]
        n140 = local read "ChnParam2write"() -> (w372:T5)
        n141 = call-dynamic "Write ChnParameter.vi"("error in (no error)"=w371, "ChnParemater"=w372, "BME_DG_Chnl in"=w373) -> ("error out"=w367:errorcluster, "BME_DG_Chnl out"=w368:refnum<class "BME_DG_Chnl.lvclass">)  [unwired: 7 in]
        n142 = call-dynamic "ModifyChnlHW.vi"("error in (no error)"=w367, "BME_DG_Chnl in"=w368) -> ("error out"=w365:errorcluster, "BME_DG_Chnl out"=w366:refnum<class "BME_DG_Chnl.lvclass">)  [unwired: 8 in]
        n143 = call "Write Chnl.vi"("error in (no error)"=w365, "BME_DG_Chnl.lvclass"=w366, "BME_DG_System in"=w370) -> ("error out"=w364:errorcluster, "BME_DG_System out"=w369:refnum<class "BME_DG_System.lvclass">)  [unwired: 7 in]
        n144 = Enqueue Element(queue=w385, element=w369, error in (no error)=w382) -> (queue out=w380:refnum<queue>, error out=w381:errorcluster)  [unwired: 1 in, 1 out]
      }
    }
    "error out" <- w158
  }
  n145 = while {
    tunnel: w33 -> [w393]
    shift-right: [w391] -> w56
    shift-left: w32 -> [w392]
    shift-right: [w388] -> w40
    shift-left: w24 -> [w390]
    tunnel: w43 -> [w387]
    tunnel: w42 -> [w386]
    stop <- w395 stop-if-true
    n146 = case shown="True" "ReadStatus" {
      tunnel: w393 -> [_ w424]
      tunnel: w392 -> [w398 w423]
      tunnel: [w398 w422] -> w391
      tunnel: w390 -> [w397 w420]
      tunnel: [w397 w406] -> w388
      tunnel: w387 -> [_ w410]
      tunnel: w386 -> [_ w409]
      frame #0 {
        n147 = Wait Until Next ms Multiple(millisecond multiple=u32 200) -> ()  [unwired: 1 out]
      }
      frame #1 {
        n148 = Dequeue Element(queue=w424, error in (no error)=w423) -> (queue out=w425:refnum<queue>, element=w421:refnum<class "BME_DG_System.lvclass">, error out=w426:errorcluster)  [unwired: 1 in, 1 out]
        n149 = Wait Until Next ms Multiple(millisecond multiple=u32 10) -> ()  [unwired: 1 out]
        n150 = call "ReadHWState.vi"("error in (no error)"=w420, "BME_DG_System in"=w421) -> ("error out"=w419:errorcluster, "Interrupts"=w415:u32[], "BME_DG_System out"=w418:refnum<class "BME_DG_System.lvclass">)  [unwired: 7 in]
        n151 = Or(x=u32 8192, y=w415) -> (x .or. y?=→"Interrupts":u32[])
        n152 = call "Read TriggersTillShot.vi"("error in (no error)"=w419, "BME_DG_System in"=w418) -> ("error out"=w411:errorcluster, "TriggerCounters"=→"TriggerCounters":i32[], "RemainingTriggers"=w417:T6, "BME_DG_System out"=w412:refnum<class "BME_DG_System.lvclass">)  [unwired: 6 in]
        n153 = call "CountsTillNextCommonTrigger.vi"("error in (no error)"=w411, "BME_DG_System in"=w412) -> ("error out"=w408:errorcluster, "LeastCommonMult"=w403:i32, "CountsRemains"=w404:i32, "BME_DG_System out"=w407:refnum<class "BME_DG_System.lvclass">)  [unwired: 6 in]
        "CountsRemains" <- w404
        n154 = Transpose 2D Array(2D array=w417) -> (transposed array=→"RemainingTriggers":T6)
        n155 = Equal?(x=w404, y=w403) -> (x = y?=w402:bool)
        n156 = case shown="No Error" w408 {
          selector: w408 -> [w430 w443]
          tunnel: w410 -> [w433 _]
          tunnel: w409 -> [w432 _]
          tunnel: w407 -> [w431 w444]
          tunnel: [w429 w443] -> w406
          tunnel: [w428 w444] -> w405
          tunnel: w402 -> [w427 _]
          frame #0 {
            n157 = case shown="True" w427 {
              tunnel: w433 -> [_ w442]
              tunnel: w432 -> [_ w441]
              tunnel: w431 -> [w435 w440]
              tunnel: w430 -> [w434 w438]
              tunnel: [w434 w437] -> w429
              tunnel: [w435 w436] -> w428
              frame #0 {
              }
              frame #1 {
                n158 = Flush Queue(queue=w442, error in (no error)=w441) -> (remaining elements=w439:T4[])  [unwired: 2 out]
                n159 = call "Update Chnls.vi"("error in (no error)"=w438, "ChnlSettings"=w439, "BME_DG_System in"=w440) -> ("error out"=w437:errorcluster, "BME_DG_System out"=w436:refnum<class "BME_DG_System.lvclass">)  [unwired: 7 in]
              }
            }
          }
          frame #1 {
          }
        }
        n160 = Enqueue Element(queue=w425, element=w405, error in (no error)=w426) -> (error out=w422:errorcluster)  [unwired: 1 in, 2 out]
      }
    }
    n161 = Unbundle By Name(w388) -> ("status"=w394:bool)
    n162 = Or(x=w394, y="stop 2") -> (x .or. y?=w395:bool)
  }
  n163 = while {
    tunnel: w33 -> [w449]
    shift-right: [w446] -> w30
    shift-left: w32 -> [w448]
    stop <- w451 stop-if-true
    n164 = case shown="True" "Aknowledge interrupts" {
      tunnel: w449 -> [_ w461]
      tunnel: w448 -> [w453 w460]
      tunnel: [w453 w459] -> w446
      frame #0 {
      }
      frame #1 {
        n165 = Dequeue Element(queue=w461, error in (no error)=w460) -> (queue out=w458:refnum<queue>, element=w457:refnum<class "BME_DG_System.lvclass">, error out=w456:errorcluster)  [unwired: 1 in, 1 out]
        n166 = call "AcknowledgeInterrupts.vi"("error in (no error)"=w456, "BME_DG_System in"=w457) -> ("error out"=w454:errorcluster, "BME_DG_System out"=w455:refnum<class "BME_DG_System.lvclass">)  [unwired: 8 in]
        n167 = Enqueue Element(queue=w458, element=w455, error in (no error)=w454) -> (error out=w459:errorcluster)  [unwired: 1 in, 2 out]
      }
    }
    n168 = Wait Until Next ms Multiple(millisecond multiple=u32 500) -> ()  [unwired: 1 out]
    n169 = Unbundle By Name(w446) -> ("status"=w450:bool)
    n170 = Or(x=w450, y="stop 3") -> (x .or. y?=w451:bool)
  }
  n171 = call <vilib>:"Merge Errors.vi"("error in 3 (no error)"=w30, "error in 2 (no error)"=w56, "error in 1 (no error)"=w57) -> ("error out"=w58:errorcluster)  [unwired: 4 in]
  n172 = call <vilib>:"Merge Errors.vi"("error in 2 (no error)"=w40, "error in 1 (no error)"=w41) -> ("error out"=w39:errorcluster)  [unwired: 5 in]
  n173 = Release Queue(queue=w45, force destroy? (F)=TRUE, error in (no error)=w39) -> (error out=w8:errorcluster)  [unwired: 2 out]
  n174 = Release Queue(queue=w59, error in (no error)=w58) -> (error out=w9:errorcluster)  [unwired: 1 in, 2 out]
  n175 = call <vilib>:"Clear Errors.vi"("error in (no error)"=w8) -> ()  [unwired: 6 in, 1 out]
  n176 = call <vilib>:"Clear Errors.vi"("error in (no error)"=w9) -> ()  [unwired: 6 in, 1 out]
